vi "Remove Null Character.vi"(11 "String":string) -> (3 "String 2":string)   [LabVIEW 2017]
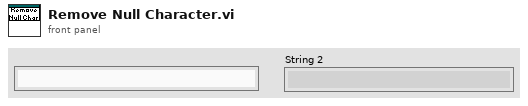
[diagram p1: front panel]
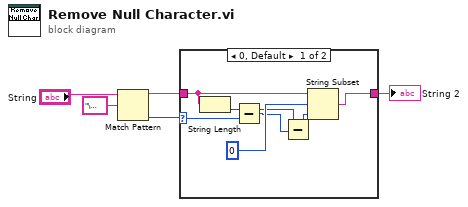
[diagram p0: block diagram]
diagram:
  n1 = Match Pattern(string="String", regular expression="\u0000") -> (before substring=w2:string, offset past match=w3:i32)  [unwired: 1 in, 2 out]
  n2 = case shown="0, Default" w3 {
    selector: w3 -> [w10 _]
    tunnel: [w11 w13] -> w1
    tunnel: w2 -> [w12 w13]
    frame 0, Default {
      n3 = String Length(string=w12) -> (length=w8:i32)
      n4 = Subtract(x=w8, y=w10) -> (x-y=w7:i32)
      n5 = Subtract(x=w8, y=w7) -> (x-y=w6:i32)
      n6 = String Subset(string=w12, offset (0)=0, length (rest)=w6) -> (substring=w11:string)
    }
    frame -1 {
    }
  }
  "String 2" <- w1
